vi "TVEMePe.vi"(8 "error in (no error)":errorcluster, 10 "Fluke":dbl[][](array[numeric]), 11 "NIST":dbl[][](array[numeric])) -> (0 "error out":errorcluster, 3 "TVEMePe":dbl[][](array[numeric]))   [LabVIEW 2014]
uses:
  <vilib>/Analysis/coordinate.llb/Angle Units.ctl
  <vilib>/Analysis/coordinate.llb/Angle Range (Degree).ctl
  <vilib>/Analysis/coordinate.llb/Wrap Angle (scalar).vi
  <vilib>/Analysis/NI_AAL_Angle.lvlib
panel:
  out "Waveform Chart":dbl[][](graph)
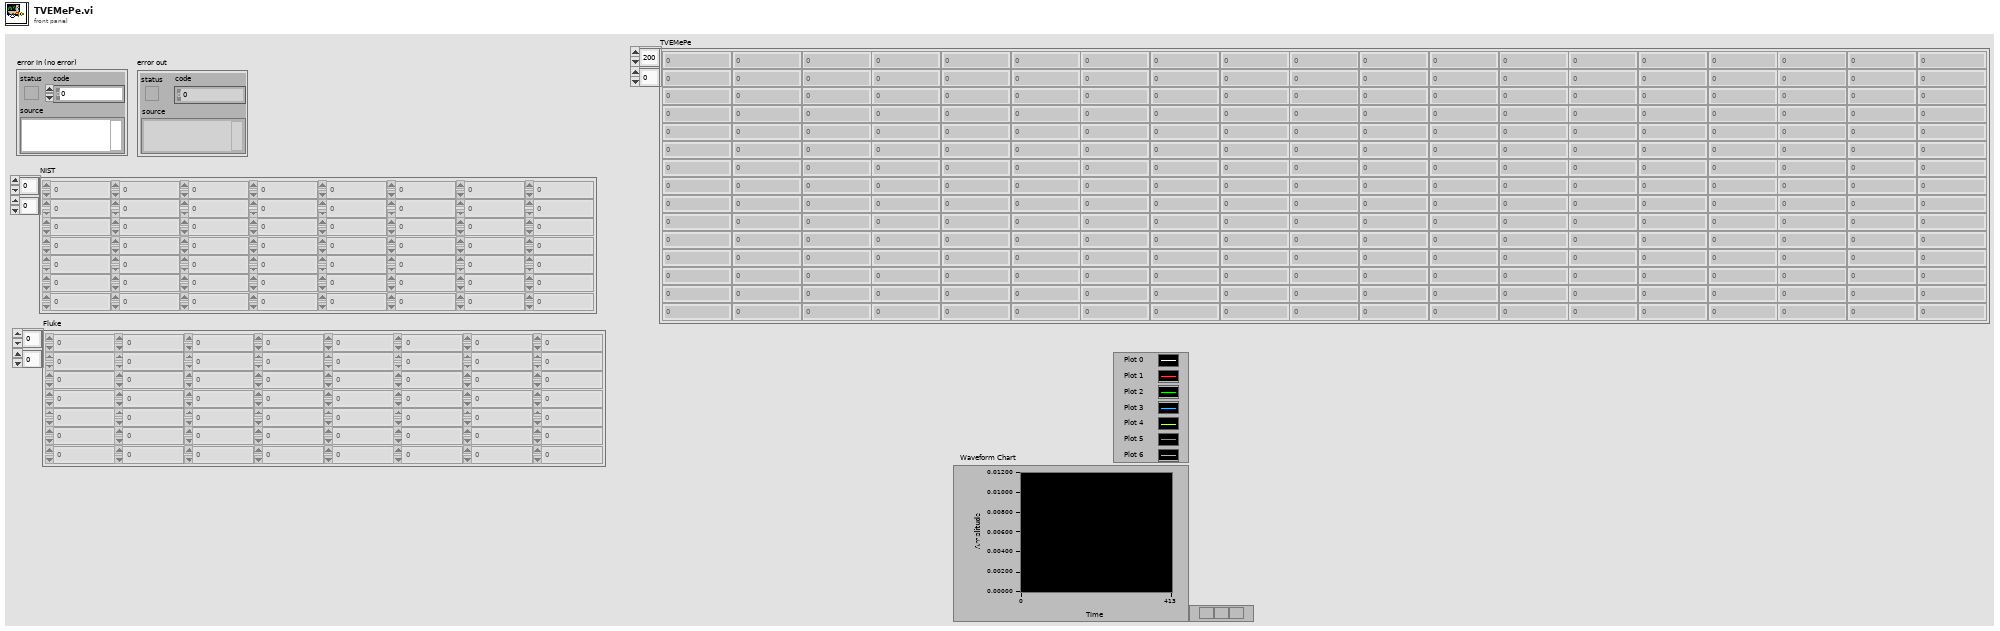
[diagram p1: front panel]
types:
  T1 = typedef "NI_AAL_Angle.lvlib/Angle Range (Degree).ctl" = u16
  T2 = typedef "NI_AAL_Angle.lvlib/Angle Units.ctl" = i32
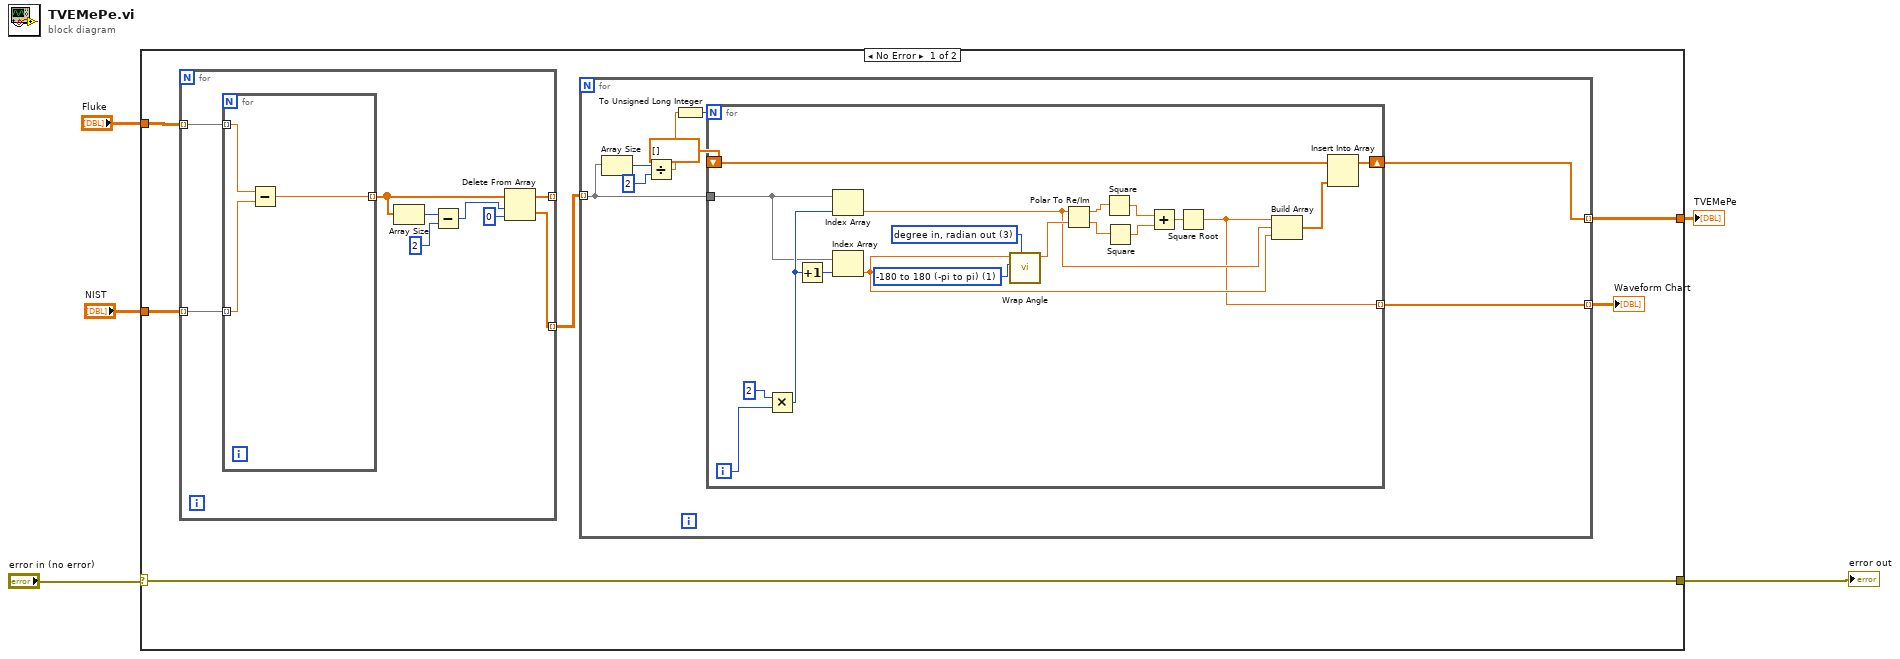
[diagram p0: block diagram]
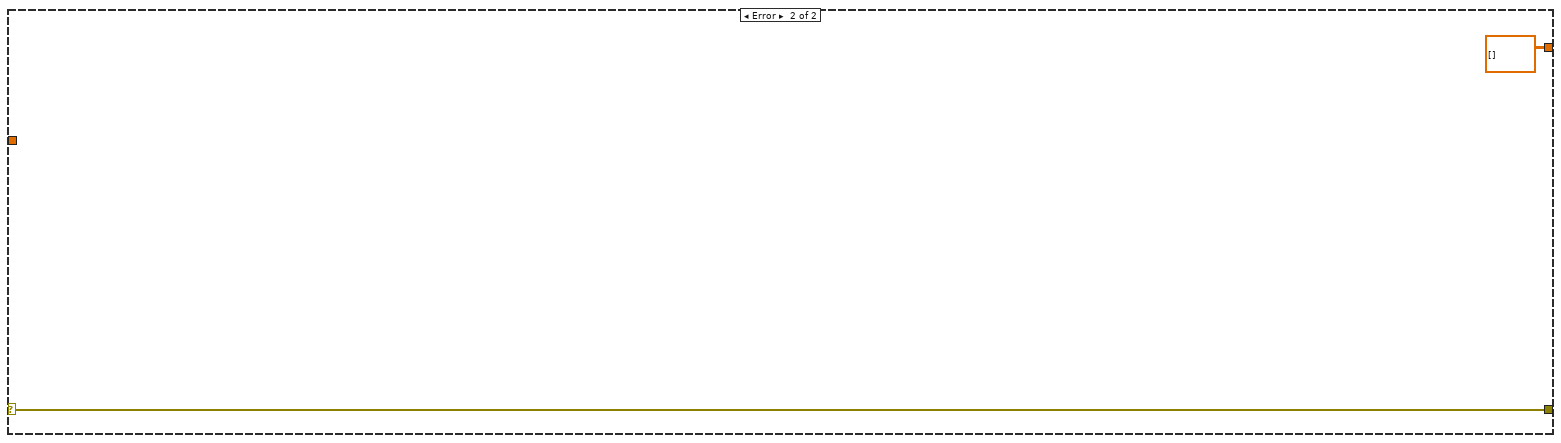
[diagram p2: hidden frame]
diagram:
  n1 = case shown="No Error" "error in (no error)" {
    selector: "error in (no error)" -> [w9 w52]
    tunnel: [w9 w52] -> w4
    tunnel: "NIST" -> [w11 _]
    tunnel: "Fluke" -> [w10 _]
    tunnel: [w7 dbl[][] []] -> w1
    frame No Error {
      n2 = for {
        tunnel: w11 -> [w47] mode=indexing
        tunnel: w10 -> [w46] mode=indexing
        tunnel: [w40] -> _ mode=indexing
        tunnel: [w39] -> w8 mode=indexing
        n3 = for {
          tunnel: w47 -> [w49] mode=indexing
          tunnel: w46 -> [w50] mode=indexing
          tunnel: [w48] -> w45 mode=indexing
          n4 = Subtract(x=w50, y=w49) -> (x-y=w48:dbl)
        }
        n5 = Array Size(array=w45) -> (size(s)=w43:i32)
        n6 = Subtract(x=w43, y=2) -> (x-y=w41:i32)
        n7 = Delete From Array(array=w45, length=w41, index=0) -> (deleted portion=w39:dbl[], array with subset deleted=w40:dbl[])
      }
      n8 = for {
        tunnel: w8 -> [w19] mode=indexing
        tunnel: [w14] -> w7 mode=indexing
        tunnel: [w12] -> w6 mode=indexing
        n9 = Array Size(array=w19) -> (size(s)=w18:i32)
        n10 = Divide(x=w18, y=2) -> (x/y=w15:dbl)
        n11 = To Unsigned Long Integer(number=w15) -> (unsigned 32bit integer=w16:u32)
        n12 = for {
          N: w16 -> [_]
          tunnel: w19 -> [w32]
          shift-right: [w30] -> w14
          shift-left: dbl[] [] -> [w28]
          tunnel: [w20] -> w12 mode=indexing
          i -> [w31]
          w34 = T1 1 items=["none", "-180 to 180 (-pi to pi)", "0 to 360 (0 to 2pi)"] ("angle range")
          w35 = T2 3 items=["radian in, radian out", "radian in, degree out", "degree in, degree out", "degree in, radian out"] ("angle units")
          n13 = Multiply(x=2, y=w31) -> (x*y=w36:i32)
          n14 = Increment(x=w36) -> (x+1=w37:i32)
          n15 = Index Array(array=w32, index=w36) -> (element=w21:dbl)
          n16 = Index Array(array=w32, index=w37) -> (element=w22:dbl)
          n17 = call-poly <vilib>:"Wrap Angle.vi"("angle units"=w35, "angle range"=w34, "angle in"=w22) -> ("angle out"=w25:dbl)  [unwired: 7 in, 1 out]
          n18 = Polar To Re/Im(2:w25, 3:w21) -> (0:w26:dbl, 1:w27:dbl)
          n19 = Square(x=w27) -> (x^2=w23:dbl)
          n20 = Square(x=w26) -> (x^2=w24:dbl)
          n21 = Add(x=w23, y=w24) -> (x+y=w33:dbl)
          n22 = Square Root(x=w33) -> (sqrt(x)=w20:dbl)
          n23 = Build Array(w20, w21, w22) -> (w29:dbl[])
          n24 = Insert Into Array(array=w28, new element=w29) -> (w30:dbl[])  [unwired: 1 in]
        }
      }
      "Waveform Chart" <- w6
    }
    frame Error {
    }
  }
  "error out" <- w4
  "TVEMePe" <- w1
